vi "Digital Input - 1 Channel - N Sample.vi"() -> ()   [LabVIEW 2019]
uses:
  <vilib>/myRIO/Instrument Drivers/Onboard IO/DI Block/typedefs/DI Block Reference.ctl
  <vilib>/myRIO/Common/Instrument Driver Framework/Utilities/typedefs/myRIO Generic Hardware Reference.ctl
  <vilib>/myRIO/Common/Instrument Driver Framework/Utilities/typedefs/Hardware Version Enum.ctl
  <vilib>/myRIO/Common/Instrument Driver Framework/Utilities/typedefs/myRIO v1.0 Reference.ctl
  <vilib>/myRIO/Common/Instrument Driver Framework/Utilities/typedefs/Generic FPGA Reference.ctl
  <vilib>/myRIO/Common/Instrument Driver Framework/myRIO v1.0/DI Block/typedefs/DI Block Channels List.ctl
  <vilib>/myRIO/Common/Instrument Driver Framework/myRIO v1.0/DI Block/typedefs/DI Block Channels Enum.ctl
  <vilib>/userdefined/High Color/nirio_resource_hc.ctl
  <vilib>/myRIO/Common/Instrument Driver Framework/ELVIS III v1.0/DI Block/vis/ELVIS III v1.1 Open DI (N Samples).vi
  <vilib>/myRIO/Common/Instrument Driver Framework/Utilities/vis/Validate Channels.vi
  <vilib>/myRIO/Common/Instrument Driver Framework/ELVIS III v1.0/Resource Manager/vis/ELVIS III v1.0 Check For Different Banks.vi
  <vilib>/myRIO/Common/Instrument Driver Framework/ELVIS III v1.0/DI Block/vis/ELVIS III v1.0 DI Block Read.vi
  <vilib>/myRIO/Common/Instrument Driver Framework/ELVIS III v1.0/DI Block/vis/ELVIS III v1.0 Close DI Block.vi
  <vilib>/myRIO/Common/Instrument Driver Framework/myRIO v1.0/UART/vis/myRIO v1.0 Close UART.vi
  <vilib>/myRIO/Common/Instrument Driver Framework/Utilities/vis/Sample Rate To Ticks.vi
  <vilib>/myRIO/Common/Instrument Driver Framework/ELVIS III v1.0/DI Block/vis/ELVIS III v1.0 Unreserve DI Block.vi
  <vilib>/myRIO/Common/Instrument Driver Framework/ELVIS III v1.0/DI Block/vis/ELVIS III v1.0 Build MUX Configuration DI Block.vi
  <vilib>/myRIO/Common/Instrument Driver Framework/ELVIS III v1.0/Resource Manager/vis/ELVIS III v1.0 Create Configuration List.vi
  <vilib>/Utility/VariantDataType/GetNumericInfo.vi
  <vilib>/Utility/error.llb/Error Cluster From Error Code.vi
  <vilib>/myRIO/Common/Instrument Driver Framework/ELVIS III v1.0/ELVIS III v1.1 Open.vi
  <vilib>/myRIO/Common/Instrument Driver Framework/ELVIS III v1.0/DI Block/vis/ELVIS III v1.0 Reserve DI Block.vi
  <vilib>/myRIO/Common/Instrument Driver Framework/ELVIS III v1.0/Resource Manager/vis/ELVIS III v1.0 Configure DMAs.vi
  <vilib>/myRIO/Common/Instrument Driver Framework/myRIO v1.0/myRIO v1.0 Close.vi
  <vilib>/myRIO/Common/Instrument Driver Framework/myRIO v1.0/Resource Manager/vis/myRIO v1.0 Block Write Configuration.vi
  <vilib>/myRIO/Common/Instrument Driver Framework/ELVIS III v1.0/DI Block/vis/ELVIS III v1.0 DI Block Read Bank B.vi
  <vilib>/myRIO/Common/Instrument Driver Framework/ELVIS III v1.0/DI Block/vis/ELVIS III v1.0 DI Block Read Bank A.vi
  <vilib>/Waveform/DWDTOps.llb/DWDT Boolean Array to Digital.vi
  <vilib>/myRIO/Common/Instrument Driver Framework/ELVIS III v1.0/Resource Manager/vis/ELVIS III v1.0 Configure IO.vi
  <vilib>/myRIO/Common/Instrument Driver Framework/ELVIS III v1.0/Resource Manager/vis/ELVIS III v1.0 Configure DI Mode.vi
  <vilib>/myRIO/Common/Instrument Driver Framework/ELVIS III v1.0/Resource Manager/vis/ELVIS III v1.0 Unreserve Channel List.vi
  <vilib>/myRIO/Common/Instrument Driver Framework/Utilities/vis/FPGA Ref Manager.vi
  <vilib>/myRIO/Common/Instrument Driver Framework/ELVIS III v1.0/ELVIS III v1.0 Reset FPGA.vi
  <vilib>/myRIO/Common/Instrument Driver Framework/myRIO v1.0/IRQ/vis/myRIO v1.0 IRQ Info FGV.vi
  <vilib>/myRIO/Common/Instrument Driver Framework/myRIO v1.0/IRQ/vis/myRIO v1.0 Timer IRQ Info FGV.vi
  <vilib>/myRIO/Common/Instrument Driver Framework/myRIO v1.0/IRQ/vis/myRIO v1.0 ISR Agent.vi
  <vilib>/myRIO/Instrument Drivers/Utilities/vis/Reset Index.vi
  <vilib>/myRIO/Common/Instrument Driver Framework/myRIO v1.0/Resource Manager/vis/myRIO v1.0 Block Write Resource Manager.vi
  <vilib>/myRIO/Instrument Drivers/Onboard IO/DI Block/vis/myRIO DI N Samples Open.xnode
  <vilib>/myRIO/Instrument Drivers/Utilities/Utilities.lvlib
  <vilib>/myRIO/Instrument Drivers/Onboard IO/DI Block/DI Block.lvlib
panel:
  out "A/DIO0":digitalwaveform(graph)
  in  "Stop":bool
  # "ELVIS III Control IO"
  # "数字输入单通道"
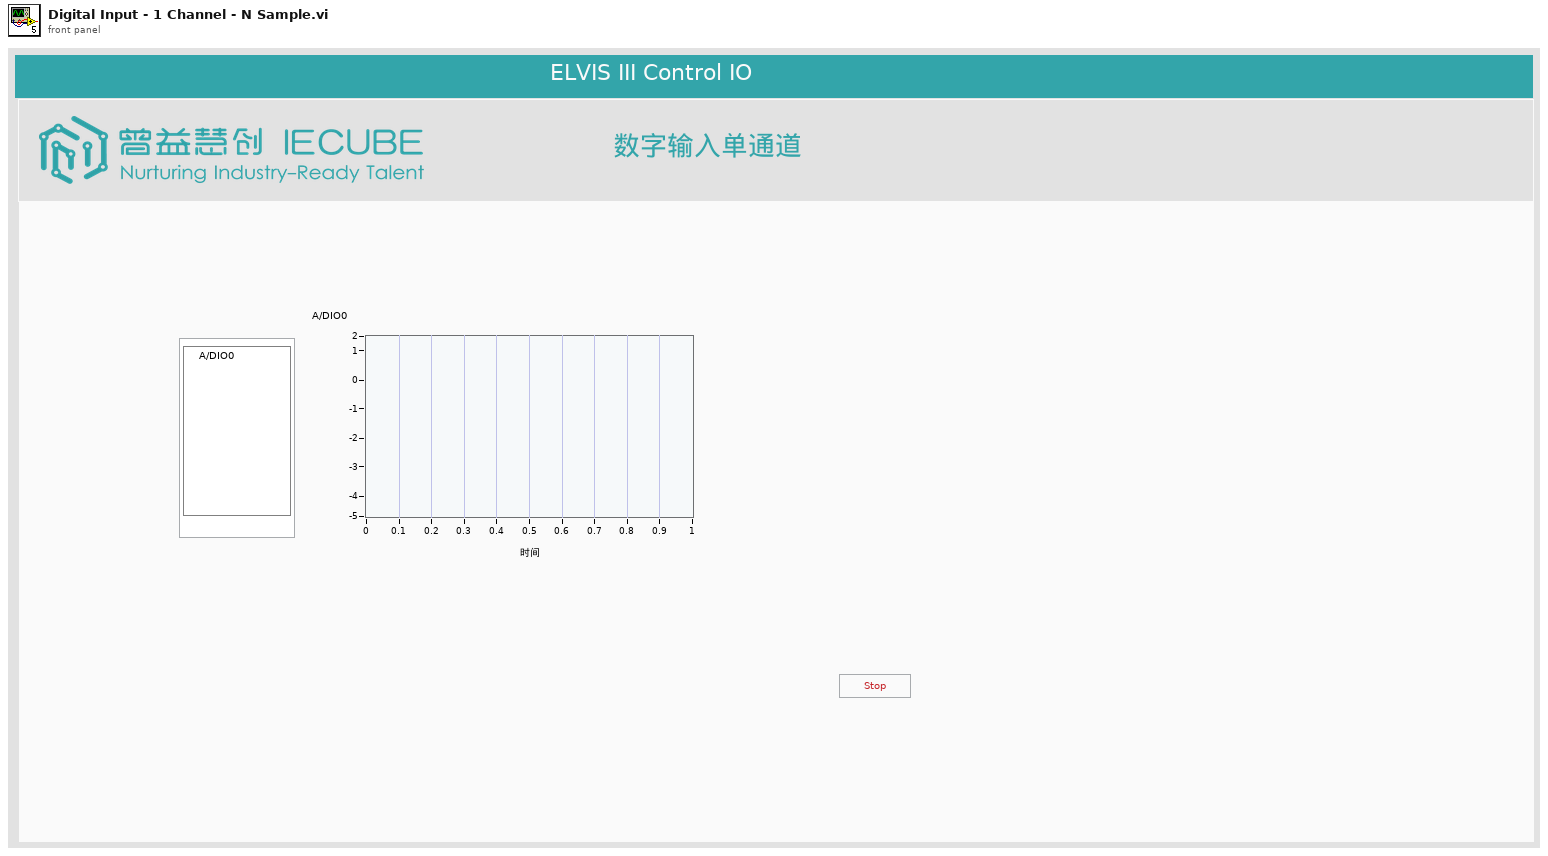
[diagram p1: front panel]
types:
  T1 = typedef "nirio_resource_hc.ctl" = tag
  T2 = typedef "Hardware Version Enum.ctl" = enum16{"Unknown", "myRIO-1900", "myRIO-1950", "roboRIO", "NI ELVIS RIO CM", "ELVIS III"}
  T3 = typedef "DI Block.lvlib/DI Block Reference.ctl" = cluster{"myRIO Reference":T4, "DI (N Samples) Channels List":T7}
  T4 = typedef "myRIO Generic Hardware Reference.ctl" = cluster{"myRIO Model":T2, "myRIO Hardware Reference":T5}
  T5 = typedef "myRIO v1.0 Reference.ctl" = cluster{"Generic FPGA Reference":T6, "Allow multiple opens":bool}
  T6 = typedef "Generic FPGA Reference.ctl" = refnum<k20>
  T7 = typedef "DI Block Channels List.ctl" = T8[]
  T8 = typedef "DI Block Channels Enum.ctl" = enum16{"Not Connected", "A/DI0 (N Samples)", "A/DI1 (N Samples)", "A/DI2 (N Samples)", "A/DI3 (N Samples)", "A/DI4 (N Samples)", "A/DI5 (N Samples)", "A/DI6 (N Samples)", "A/DI7 (N Samples)", "A/DI8 (N Samples)", "A/DI9 (N Samples)", "A/DI10 (N Samples)", "A/DI11 (N Samples)", "A/DI12 (N Samples)", "A/DI13 (N Samples)", "A/DI14 (N Samples)", "A/DI15 (N Samples)", "A/DI16 (N Samples)", "A/DI17 (N Samples)", "A/DI18 (N Samples)", "A/DI19 (N Samples)", "B/DI0 (N Samples)", "B/DI1 (N Samples)", "B/DI2 (N Samples)", "B/DI3 (N Samples)", "B/DI4 (N Samples)", "B/DI5 (N Samples)", "B/DI6 (N Samples)", "B/DI7 (N Samples)", "B/DI8 (N Samples)", "B/DI9 (N Samples)", "B/DI10 (N Samples)", "B/DI11 (N Samples)", "B/DI12 (N Samples)", "B/DI13 (N Samples)", "B/DI14 (N Samples)", "B/DI15 (N Samples)", "B/DI16 (N Samples)", "B/DI17 (N Samples)", "B/DI18 (N Samples)", "B/DI19 (N Samples)"}
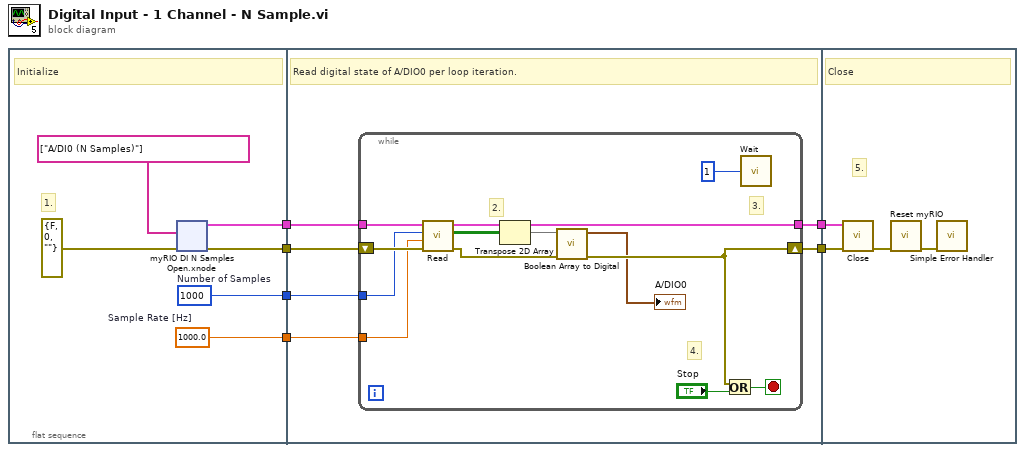
[diagram p0: block diagram]
diagram:
  n1 = flat-sequence {
    tunnel: [w11] -> w6
    tunnel: [w10] -> w5
    tunnel: [w8] -> w2
    tunnel: [w7] -> w1
    tunnel: [w34] -> w4
    tunnel: w6 -> [w33]
    tunnel: w5 -> [w32]
    tunnel: [w31] -> w3
    tunnel: w2 -> [w30]
    tunnel: w1 -> [w29]
    tunnel: w4 -> [w50]
    tunnel: w3 -> [w48]
    frame #0 {
      w7 = u32 1000  # Number of Samples
      w8 = 1000.0  # Sample Rate [Hz]
      # "1."
      # "Initialize"
      n2 = xnode "myRIO DI N Samples Open.xnode"("error in (no error)"=errorcluster {"status"=FALSE, "code"=0, "source"=""} ("Error In"), "Channel Names"=tag[] ["A/DI0 (N Samples)"]) -> ("error out"=w11:errorcluster, "DI (N Samples) Ref Out"=w10:T3)  [unwired: 1 in]
    }
    frame #1 {
      # "Read digital state of A/DIO0 per loop iteration."
      n3 = while {
        shift-right: [w38] -> w34
        shift-left: w33 -> [w44]
        tunnel: w32 -> [w42]
        tunnel: [w43] -> w31
        tunnel: w30 -> [w41]
        tunnel: w29 -> [w40]
        stop <- w45 stop-if-true
        # "4."
        # "3."
        # "2."
        n4 = call <vilib>:"Read.vi"("error in (no error)"=w44, "Sample Rate [Hz]"=w41, "Number of Samples"=w40, "DI (N Samples) Ref In"=w42) -> ("error out"=w39:errorcluster, "Values"=w37:bool[][], "DI (N Samples) Ref Out"=w43:T3)  [unwired: 5 in]
        n5 = Transpose 2D Array(2D array=w37) -> (transposed array=w36:bool[][])
        n6 = call-poly <vilib>:"Boolean Array to Digital.vi"("error in (no error)"=w39, "boolean array"=w36) -> ("error out"=w38:errorcluster, "digital waveform"=→"A/DIO0":digitalwaveform)  [unwired: 8 in]
        n7 = Or(x=w38, y="Stop") -> (x .or. y?=w45:bool)
        n8 = call "Wait"("Count(mSec)"=u32 1 ("Count(uSec)")) -> ()  [unwired: 1 out]
      }
    }
    frame #2 {
      # "5."
      # "Close"
      n9 = call <vilib>:"Close.vi"("error in (no error)"=w50, "DI (N Samples) Ref In"=w48) -> ("error out"=w49:errorcluster)  [unwired: 9 in]
      n10 = call <vilib>:"Reset myRIO.vi"("error in (no error)"=w49) -> ("error out"=w51:errorcluster)  [unwired: 10 in]
      n11 = call <vilib>:"Simple Error Handler.vi"("error in (no error)"=w51) -> ()  [unwired: 4 in, 5 out]
    }
  }
